vi "setObstructions.vi"(8 "error in (no error)":errorcluster, 10 "Obstructions":refnum<class "Obstruction.lvclass">[](array[class]), 11 "OccupancyMap in":refnum<class "OccupancyMap.lvclass">) -> (0 "error out":errorcluster, 3 "OccupancyMap out":refnum<class "OccupancyMap.lvclass">)   [LabVIEW 2013, in "OccupancyMap.lvclass"]
uses:
  OccupancyMap.lvclass
  Obstruction/Obstruction.lvclass
  OccupancyMap.lvclass/OccupancyMap.ctl
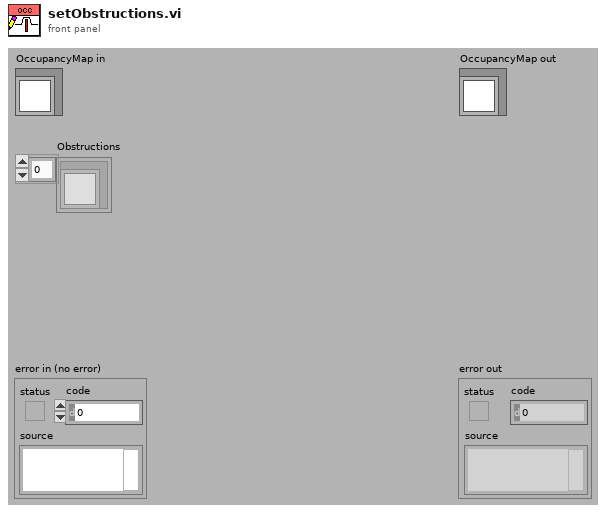
[diagram p1: front panel]
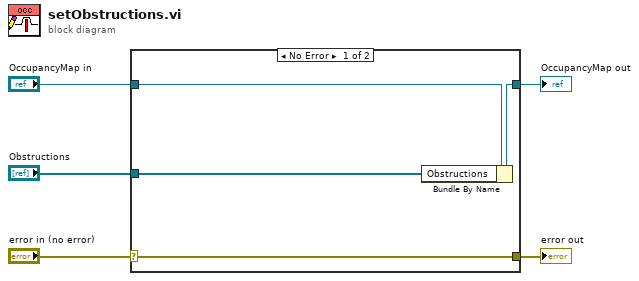
[diagram p0: block diagram]
diagram:
  n1 = case shown="No Error" "error in (no error)" {
    selector: "error in (no error)" -> [w9 w10]
    tunnel: [w9 w10] -> w4
    tunnel: [w7 w11] -> w2
    tunnel: "OccupancyMap in" -> [w8 w11]
    tunnel: "Obstructions" -> [w6 _]
    frame No Error {
      n2 = Bundle By Name(cluster=w8, "Obstructions"=w6) -> (w7:refnum<class "OccupancyMap.lvclass">)
    }
    frame Error {
    }
  }
  "error out" <- w4
  "OccupancyMap out" <- w2
